vi "ChooseSwitching.vi"(8 "error in (no error)":errorcluster, 11 "Instrument name IN":string(combo)) -> (0 "error in (no error) 2":errorcluster, 3 "Switching.lvclass":refnum<class "Switching.lvclass">)   [LabVIEW 2018, in "Switching.lvclass"]
uses:
  Switching.lvclass
  GPIBSwitching/GPIBSwitching.lvclass
  C:/ProbeTestSoftware2019/itk-strip-sensor-qc/InstrControl/Switching/Switching.lvclass
  LXIPXISwitching/LXIPXISwitching.lvclass
  InstrumentSetup.vi
  InstrControl.lvclass
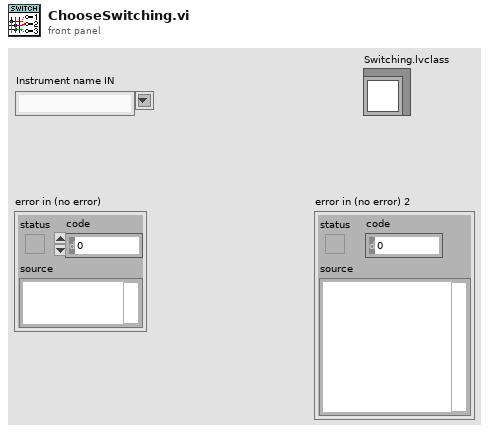
[diagram p1: front panel]
types:
  T1 = cluster{"KE 2410":cluster{"Instrument name":string, "GPIB address":string, "Instrument type":u16}, "KE 6517":cluster{"Instrument name":string, "GPIB address":string, "Instrument type":u16}, "KE 487":cluster{"Instrument name":string, "GPIB address":string, "Instrument type":u16}, "KE 2657A":cluster{"Instrument name":string, "GPIB address":string, "Instrument type":u16}, "KE 236":cluster{"Instrument name":string, "GPIB address":string, "Instrument type":u16}, "WK 6440B":cluster{"Instrument name":string, "GPIB address":string, "Instrument type":u16}, "WK 6425":cluster{"Instrument name":string, "GPIB address":string, "Instrument type":u16}, "Pickering Matrix":cluster{"Instrument name":string, "GPIB address":string, "Instrument type":u16}, "KE 2000":cluster{"Instrument name":string, "GPIB address":string, "Instrument type":u16}}
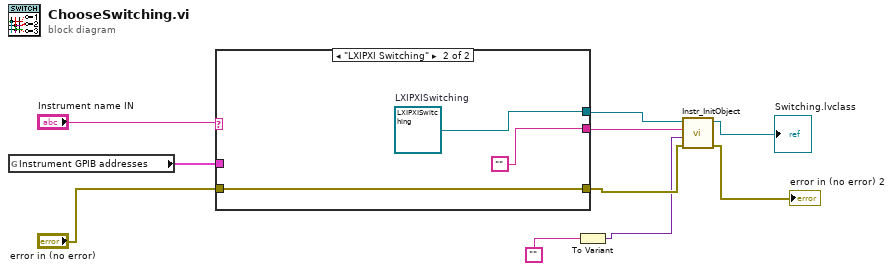
[diagram p0: block diagram]
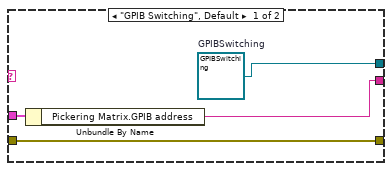
[diagram p2: hidden frame]
diagram:
  n1 = global read "InstrumentSetup.vi" "Instrument GPIB addresses"() -> (w3:T1)
  n2 = case shown="\"LXIPXI Switching\"" "Instrument name IN" {
    tunnel: "error in (no error)" -> [w14 w17]
    tunnel: [w14 w17] -> w5
    tunnel: w3 -> [w13 _]
    tunnel: [w12 ""] -> w2
    tunnel: [w11 w15] -> w1
    frame "GPIB Switching", Default {
      w11 = refnum<class "GPIBSwitching.lvclass"> refnum  # GPIBSwitching
      n3 = Unbundle By Name(w13) -> ("Pickering Matrix.GPIB address"=w12:string)
    }
    frame "LXIPXI Switching" {
      w15 = refnum<class "LXIPXISwitching.lvclass"> refnum  # LXIPXISwitching
    }
  }
  n4 = To Variant(anything="") -> (Variant=w4:variant)
  n5 = call-dynamic "Instr_InitObject.vi"("error in (no error)"=w5, "Instrument Configuration"=w4, "GPIB Address"=w2, "Switching in"=w1) -> ("error out"=→"error in (no error) 2":errorcluster, "Switching out"=→"Switching.lvclass":refnum<class "Switching.lvclass">)  [unwired: 6 in]
